vi "Set PWM Duty Cycle.vi"(0 "reference in":refnum<class "NI-DAQmx.lvclass">, 2 "PWM Duty Cycle (%)":dbl, 5 "error in (no error)":errorcluster) -> (14 "reference out":refnum<class "NI-DAQmx.lvclass">, 19 "error out":errorcluster)   [LabVIEW 2020, in "NI-DAQmx.lvclass"]
uses:
  NI-DAQmx.lvclass
  <vilib>/DAQmx/write.llb/DAQmx Write (Analog 1D DBL 1Chan NSamp).vi
  <vilib>/DAQmx/miscellaneous.llb/DAQmx Fill In Error Info.vi
  <vilib>/Analysis/NI_AALBase.lvlib
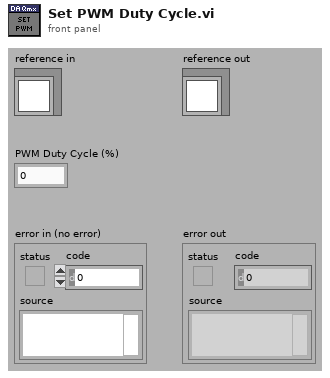
[diagram p1: front panel]
types:
  T1 = typedef "NI-DAQmx.lvclass/ObjectAttributes.ctl" = cluster{"AI Task":refnum<k21>, "DO Task":refnum<k21>, "AO Task":refnum<k21>, "Latest Values":dbl[], "Signal List":T2[], "PWM Duty Cycle (%)":dbl, "PWM Amplitude (V)":dbl, "PWM Frequency (Hz)":dbl, "DO States":bool[]}
  T2 = typedef "IO Signal List.ctl" = enum16{"Timestamp", "PSU_FB_U_VDC", "PSU_FB_I_AMP", "PSU_FB_W_WATT", "PSU_CMD_U_VDC", "PSU_CMD_I_AMP", "PSU_CMD_OUTPUT", "LCR_PRIMARY", "LCR_SECONDARY", "UV_R_Ohm", "UW_R_Ohm", "VW_R_Ohm", "UV_L_H", "UW_L_H", "VW_L_H", "U_U_VDC", "V_U_VDC", "W_U_VDC", "U_I_AMP", "V_I_AMP", "W_I_AMP", "PWM_CMD_DC_%", "PWM_CMD_VDC", "PWM_CMD_Hz", "PWM_FB_DC_%", "PWM_FB_VDC", "PWM_FB_Hz", "DO_RELAY_U_LCR_A", "DO_RELAY_V_LCR_A", "DO_RELAY_V_LCR_B", "DO_RELAY_W_LCR_B", "DIFF_UV_UW_L_H", "DIFF_UV_VW_L_H", "DIFF_UW_VW_L_H", "DIFF_UV_UW_R_Ohm", "DIFF_UV_VW_R_Ohm", "DIFF_UW_VW_R_Ohm", "DIFF_UV_U_VDC", "DIFF_UW_U_VDC", "DIFF_VW_U_VDC"}
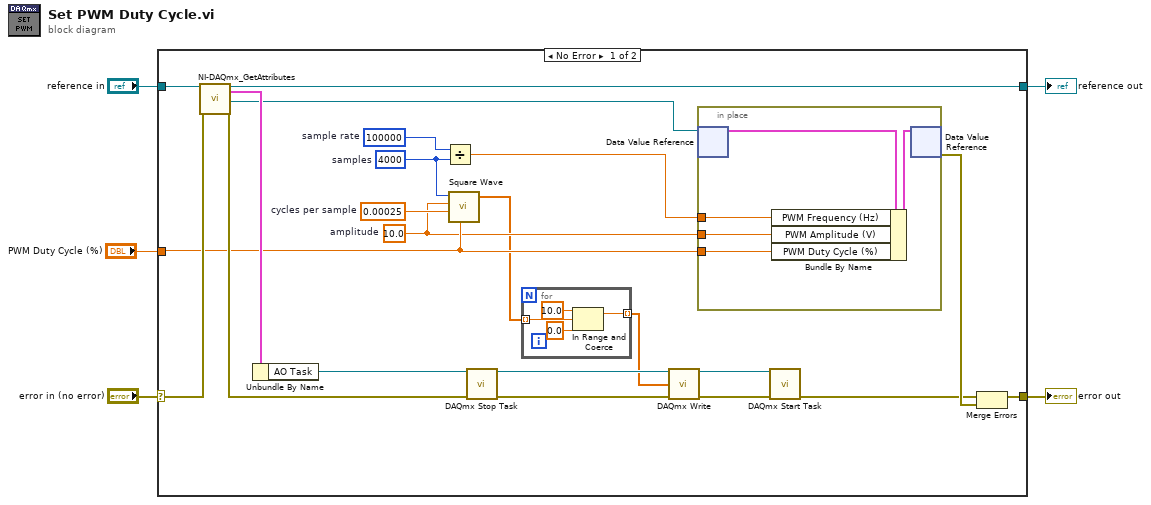
[diagram p0: block diagram]
diagram:
  n1 = case shown="No Error" "error in (no error)" {
    selector: "error in (no error)" -> [w26 w38]
    tunnel: [w22 w38] -> w4
    tunnel: [w23 w37] -> w2
    tunnel: "reference in" -> [w27 w37]
    tunnel: "PWM Duty Cycle (%)" -> [w12 _]
    frame No Error {
      w11 = 100000  # sample rate
      w9 = 10.0  # amplitude
      w13 = 0.00025  # cycles per sample
      w10 = 4000  # samples
      n2 = call "NI-DAQmx_GetAttributes.vi"("reference in"=w27, "error in (no error)"=w26) -> ("reference out"=w23:refnum<class "NI-DAQmx.lvclass">, "Data"=w25:T1, "DataRef"=w21:refnum<data-value>, "error out"=w16:errorcluster)  [unwired: 14 in]
      n3 = Unbundle By Name(w25) -> ("AO Task"=w14:refnum<k21>)
      n4 = Divide(x=w11, y=w10) -> (x/y=w8:dbl)
      n5 = call <vilib>:"Square Wave.vi"("samples"=w10, "amplitude"=w9, "frequency"=w13, "duty cycle (%)"=w12) -> ("square wave"=w6:dbl[])  [unwired: 2 in, 2 out]
      n6 = call <vilib>:"DAQmx Stop Task.vi"("task/channels in"=w14, "error in"=w16) -> ("task out"=w19:refnum<k21>, "error out"=w20:errorcluster)  [unwired: 12 in]
      n7 = for {
        tunnel: w6 -> [w31] mode=indexing
        tunnel: [w28] -> w7 mode=indexing
        n8 = In Range and Coerce(upper limit=10.0, x=w31, lower limit=0.0) -> (coerced(x)=w28:dbl)  [unwired: 1 out]
      }
      n9 = call-poly <vilib>:"DAQmx Write.vi"("task/channels in"=w19, "data"=w7, "error in"=w20) -> ("task out"=w17:refnum<k21>, "error out"=w18:errorcluster)  [unwired: 10 in, 1 out]
      n10 = in-place {
        in-place-border: w12 -> [w34]
        in-place-border: w9 -> [w33]
        in-place-border: w8 -> [w32]
        n11 = in-place-dvr #1(w21) -> (w35:T1)  [unwired: 1 out]
        n12 = Bundle By Name(cluster=w35, "PWM Frequency (Hz)"=w32, "PWM Amplitude (V)"=w33, "PWM Duty Cycle (%)"=w34) -> (w36:T1)
        n13 = in-place-dvr #1(w36) -> (w24:errorcluster)  [unwired: 1 out]
      }
      n14 = call <vilib>:"DAQmx Start Task.vi"("task/channels in"=w17, "error in"=w18) -> ("error out"=w15:errorcluster)  [unwired: 12 in, 1 out]
      n15 = Merge Errors(w15, w24) -> (w22:errorcluster)
    }
    frame Error {
    }
  }
  "error out" <- w4
  "reference out" <- w2
